vi "Camera-StartStopStream.vi"(3 "Error IN":errorcluster, 4 "Camara ON?":bool, 5 "hCamera IN":u32) -> (0 "Error OUT":errorcluster, 2 "hCamera OUT":u32)   [LabVIEW 2010]
uses:
  <vilib>/addons/PixeLINK/Low Level Functions/ACQUISITION.llb/TDPU-Acquisition-StreamState.ctl
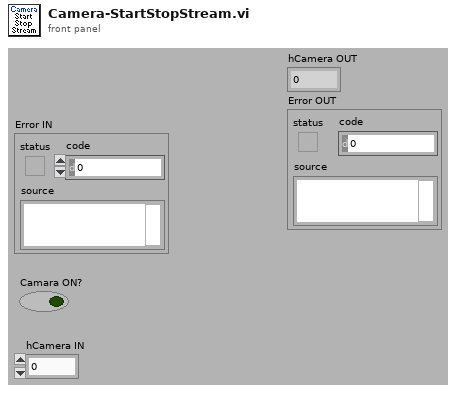
[diagram p1: front panel]
types:
  T1 = typedef "TDPU-Acquisition-StreamState.ctl" = u32
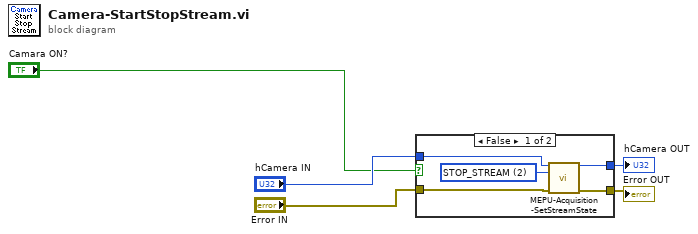
[diagram p0: block diagram]
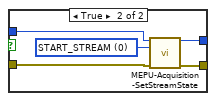
[diagram p2: hidden frame]
diagram:
  n1 = case shown="False" "Camara ON?" {
    tunnel: "hCamera IN" -> [w9 w14]
    tunnel: "Error IN" -> [w8 w13]
    tunnel: [w7 w12] -> w2
    tunnel: [w6 w11] -> w1
    frame False {
      w10 = T1 2 items=["START_STREAM", "PAUSE_STREAM", "STOP_STREAM"] ("uStreamState IN")
      n2 = call <vilib>:"MEPU-Acquisition-SetStreamState.vi"("hCamera IN"=w9, "uStreamState IN"=w10, "Error IN"=w8) -> ("hCamera OUT"=w7:u32, "Error OUT"=w6:errorcluster)  [unwired: 11 in]
    }
    frame True {
      w15 = T1 0 items=["START_STREAM", "PAUSE_STREAM", "STOP_STREAM"] ("uStreamState IN")
      n3 = call <vilib>:"MEPU-Acquisition-SetStreamState.vi"("hCamera IN"=w14, "uStreamState IN"=w15, "Error IN"=w13) -> ("hCamera OUT"=w12:u32, "Error OUT"=w11:errorcluster)  [unwired: 11 in]
    }
  }
  "hCamera OUT" <- w2
  "Error OUT" <- w1
